vi "STM-program.vi"() -> (1 "OutDir":i32, 2 "Out Speed":i32, 3 "Out Degree":dbl, 5 "Stepper Motor":string, 7 "Channels (A:B:C:D...) (Out)":string)   [LabVIEW 2015]
uses:
  Control Button/Exit.ctl
  Control PB/Next_.ctl
panel:
  in  "Servo Motor":i32[](listbox)=[0]
  in  "Speed (mm/s)":i32
  in  "Travel Distance(mm)":dbl
  in  "Motor Direction":enum16{"Direction Selection", "CW", "CCW"}(ring)
  in  "OK Button":T1
  in  "stop":T2
  # "Servo Step Program Setting Window"
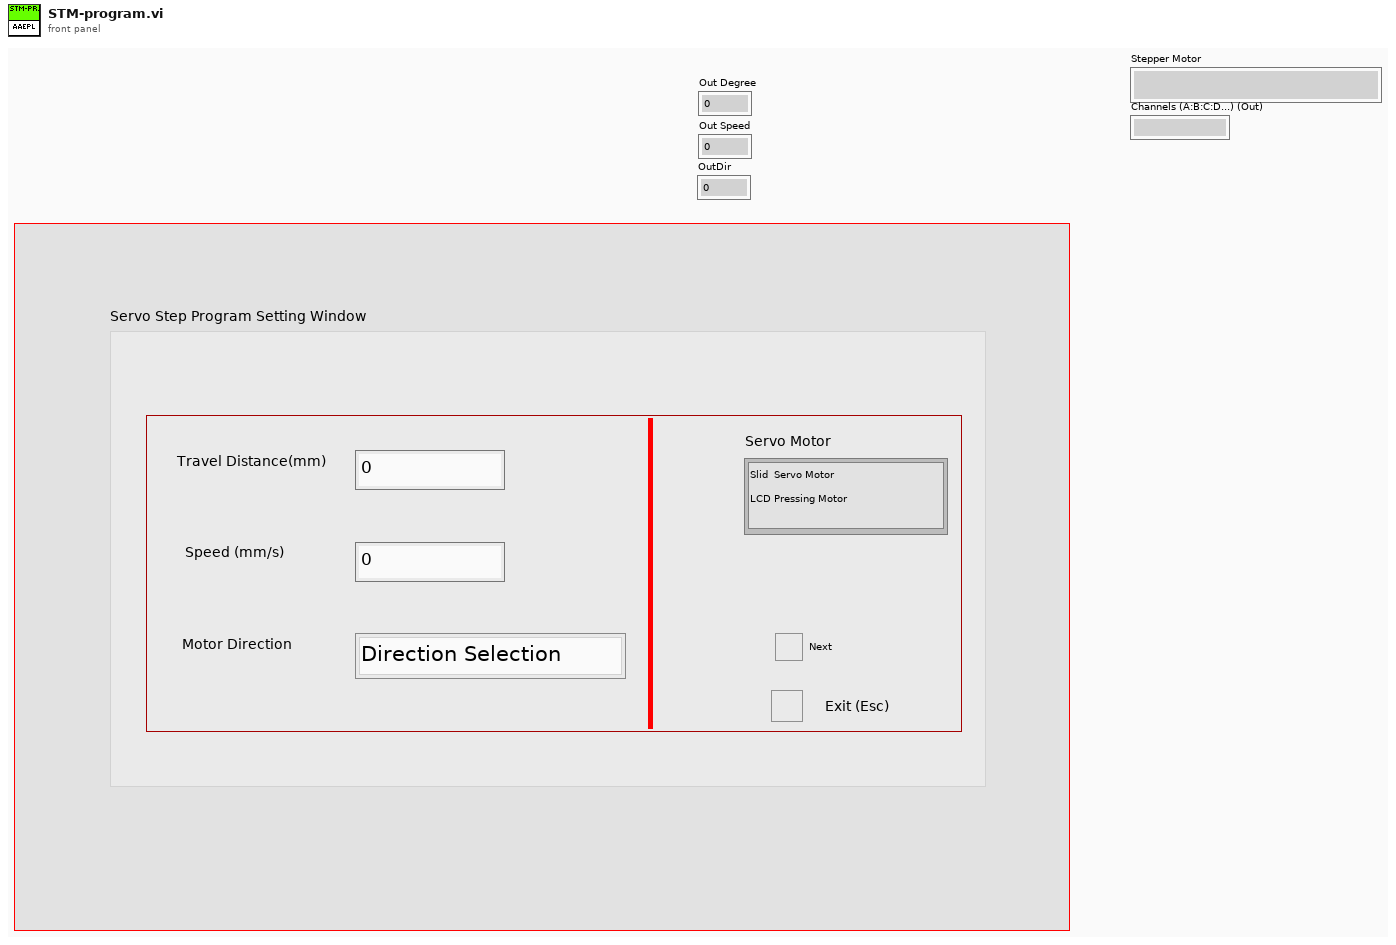
[diagram p1: front panel]
types:
  T1 = typedef "Next_.ctl" = bool
  T2 = typedef "Exit.ctl" = bool
  T3 = cluster{"Channel Type":string, "Channels":string, "Wait/Poll (ms)":u32, "Parameter":u8, "STM-Speed":u8, "STM-Degree":u32, "Direction":u8}
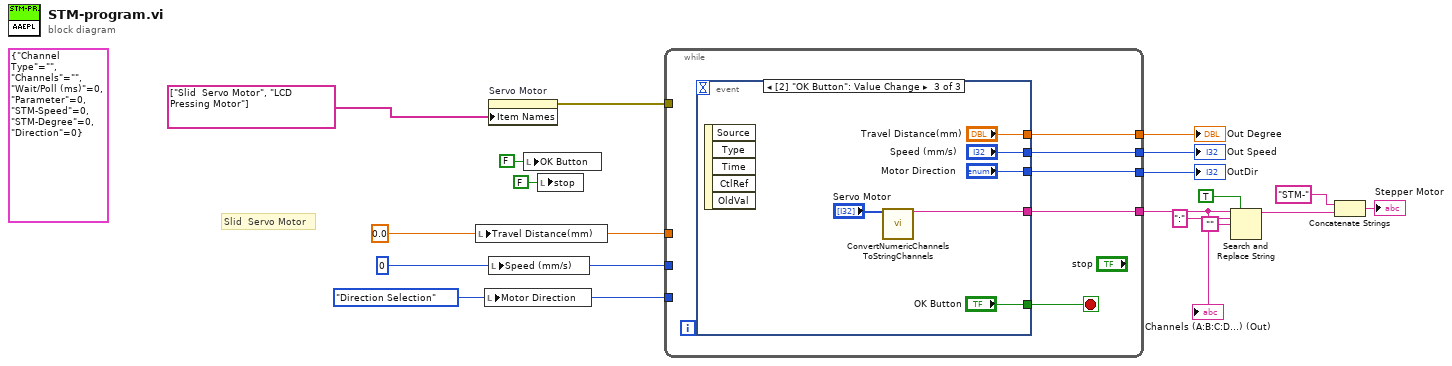
[diagram p0: block diagram]
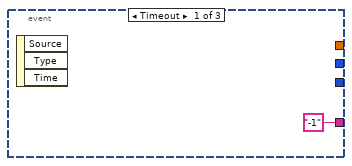
[diagram p2: hidden frame]
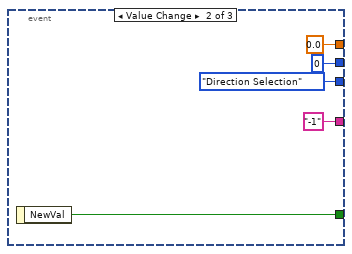
[diagram p3: hidden frame]
diagram:
  w12 = enum16{"Direction Selection", "CW", "CCW"}."Direction Selection" ("Enum")
  w13 = 0 ("Speed")
  w14 = 0.0 ("Degree")
  (unwired) T3 {"Channel Type"="", "Channels"="", "Wait/Poll (ms)"=0, "Parameter"=0, "STM-Speed"=0, "STM-Degree"=0, "Direction"=0} ("Step")
  # "Slid  Servo Motor"
  n1 = local write "Travel Distance(mm)"(w14) -> ()
  n2 = local write "Motor Direction"(w12) -> ()
  n3 = property on="Servo Motor" class="LstBox (strict)"("Item Names"=string[] ["Slid  Servo Motor", "LCD Pressing Motor"]) -> (error out=w2:errorcluster)  [unwired: 2 in, 1 out]
  n4 = local write "Speed (mm/s)"(w13) -> ()
  n5 = local write "OK Button"(T1 FALSE ("OK Button")) -> ()
  n6 = local write "stop"(FALSE ("stop")) -> ()
  n7 = while {
    tunnel: [w21] -> w17
    tunnel: [w20] -> w16
    tunnel: [w19] -> w15
    tunnel: w14 -> [_]
    tunnel: w13 -> [_]
    tunnel: w12 -> [_]
    tunnel: [w18] -> w11
    tunnel: w2 -> [_]
    stop <- w22 stop-if-true
    n8 = event shown="[2] \"OK Button\": Value Change" {
      selector: _ -> [_ _ _]
      dyn-events: _ -> [_ _ _]
      timeout: _ -> [_ _ _]
      tunnel: [_ w28 "OK Button"] -> w22
      tunnel: [_ 0.0 ("Degree") "Travel Distance(mm)"] -> w21
      tunnel: [_ 0 ("Speed") "Speed (mm/s)"] -> w20
      tunnel: [_ enum16{"Direction Selection", "CW", "CCW"}."Direction Selection" ("Enum") "Motor Direction"] -> w19
      tunnel: ["-1" ("Channels (A:B:C:D...) (Out)") "-1" ("Channels (A:B:C:D...) (Out)") w29] -> w18
      event Timeout {
        n9 = event-data() -> ()  [unwired: 1 in, 3 out]
      }
      event Value Change {
        n10 = event-data() -> ("NewVal"=w28:T2)  [unwired: 1 in]
      }
      event Value Change {
        n11 = event-data() -> ()  [unwired: 1 in, 5 out]
        n12 = call "ConvertNumericChannelsToStringChannels.vi"("Channels (In)"="Servo Motor") -> ("Channels (A:B:C:D...) (Out)"=w29:string)  [unwired: 14 in]
      }
    }
  }
  "Out Degree" <- w17
  "Out Speed" <- w16
  "OutDir" <- w15
  "Channels (A:B:C:D...) (Out)" <- w11
  n13 = Search and Replace String(replace all?=TRUE ("replace all? (F)"), input string=w11, search string=":" ("replace string (\"\")"), replace string="") -> (result string=w6:string)  [unwired: 4 in, 3 out]
  n14 = Concatenate Strings("STM-", w6) -> (→"Stepper Motor":string)
